vi "Oracle to Array.vi"(8 "error in":errorcluster, 11 "string in":string) -> (0 "error out":errorcluster, 1 "Empty?":bool, 3 "SR number array out":i32[](array[numeric]))   [LabVIEW 2018]
panel:
  out "SR List String":string
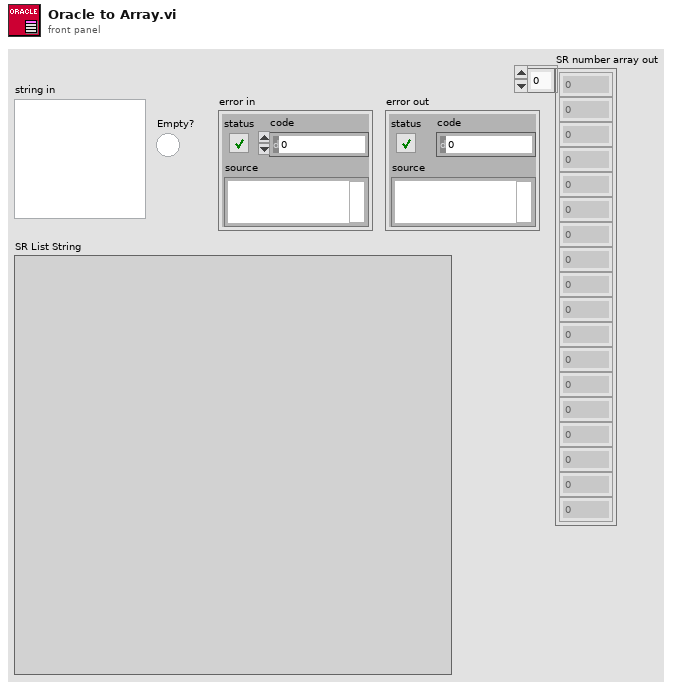
[diagram p1: front panel]
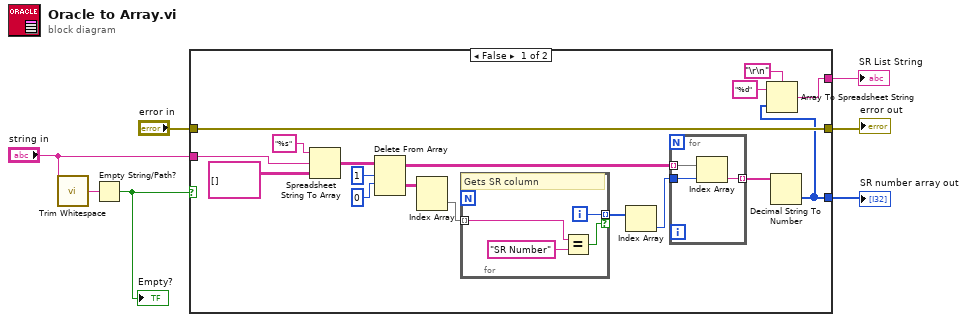
[diagram p0: block diagram]
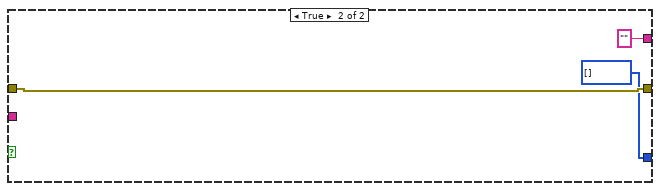
[diagram p2: hidden frame]
diagram:
  n1 = call <vilib>:"Trim Whitespace.vi"("string"="string in") -> ("trimmed string"=w7:string)  [unwired: 1 in]
  n2 = Empty String/Path?(string/path=w7) -> (empty?=w6:bool)
  "Empty?" <- w6
  n3 = case shown="False" w6 {
    tunnel: [w17 w34] -> w2
    tunnel: "string in" -> [w16 _]
    tunnel: "error in" -> [w17 w34]
    tunnel: [w8 i32[] []] -> w1
    tunnel: [w10 ""] -> w3
    frame False {
      n4 = Spreadsheet String To Array(format string="%s", spreadsheet string=w16, array type (2D Dbl)=string[][] []) -> (array=w13:string[][])  [unwired: 1 in]
      n5 = Delete From Array(array=w13, length=1, index (row)=0) -> (deleted portion=w24:string[][], array with subset deleted=w20:string[][])  [unwired: 1 in]
      n6 = Index Array(array=w24) -> (element=w23:string[])  [unwired: 2 in]
      n7 = for {
        tunnel: [w26] -> w22 mode=indexing if=w27
        tunnel: w23 -> [w25] mode=indexing
        i -> [w26]
        # "Gets SR column"
        n8 = Equal?(x=w25, y="SR Number") -> (x = y?=w27:bool)
      }
      n9 = Index Array(array=w22) -> (element=w21:i32)  [unwired: 1 in]
      n10 = for {
        tunnel: w21 -> [w30]
        tunnel: w20 -> [w31] mode=indexing
        tunnel: [w29] -> w12 mode=indexing
        n11 = Index Array(array=w31, index=w30) -> (element=w29:string)
      }
      n12 = Decimal String To Number(string=w12) -> (number=w8:i32[])  [unwired: 2 in, 1 out]
      n13 = Array To Spreadsheet String(delimiter (Tab)="\r\n", array=w8, 3:"%d" ("format string")) -> (spreadsheet string=w10:string)
    }
    frame True {
    }
  }
  "error out" <- w2
  "SR number array out" <- w1
  "SR List String" <- w3
